vi "Generate VS Channels Info.vi"(11 "Transfer Type":enum16{"Acyclic", "Scheduled"}(ring)) -> (0 "Tx Trigger Channels Array":string[](array[string]), 1 "Tx Disable Channels Array":string[](array[string]), 2 "Tx Channels Array":string[](array[string]), 3 "Rx Channels Array":string[](array[string]), 4 "Is First Parameter? Array":bool[](array[boolean]))   [LabVIEW 2020]
uses:
  b281cc4c-f5bf-4263-a2a4-b8c933cd51f6.vi
  9ae52f1a-1e4b-4aa8-8e73-03c214062afe.vi
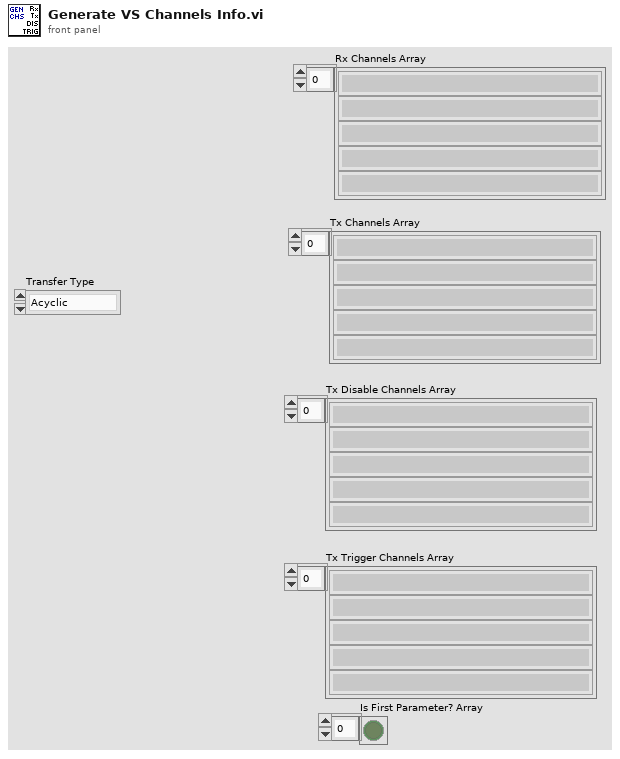
[diagram p1: front panel]
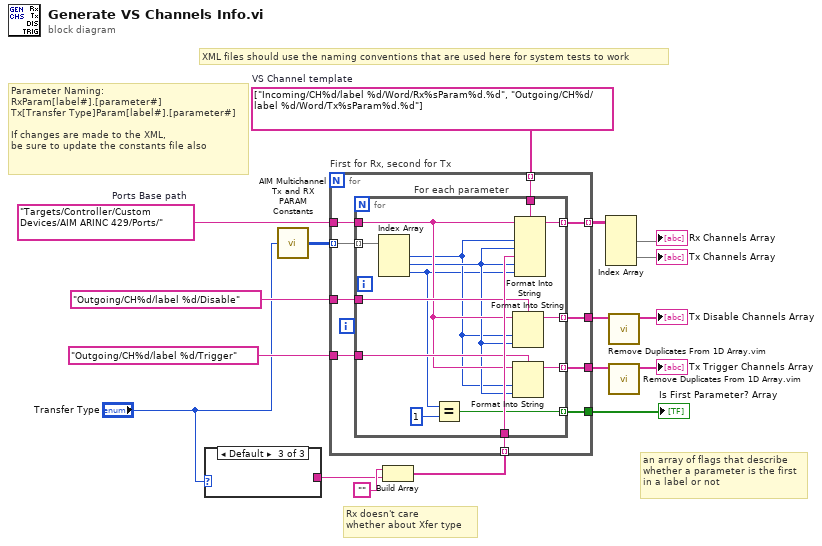
[diagram p0: block diagram]
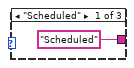
[diagram p2: hidden frame]
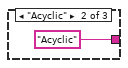
[diagram p3: hidden frame]
diagram:
  w10 = "Targets/Controller/Custom Devices/AIM ARINC 429/Ports/"  # Ports Base path
  w17 = string[] ["Incoming/CH%d/label %d/Word/Rx%sParam%d.%d", "Outgoing/CH%d/label %d/Word/Tx%sParam%d.%d"]  # VS Channel template
  # "Rx doesn't care\nwhether about Xfer type"
  # "an array of flags that describe\nwhether a parameter is the first\nin a label or not"
  # "Parameter Naming:\nRxParam[label#].[parameter#]\nTx[Transfer Type]Param[label#].[parameter#]\n\nIf changes are made to the XML,\nbe sure to update the constants file also"
  # "XML files should use the naming conventions that are used here for system tests to work"
  n1 = case shown="Default" "Transfer Type" {
    tunnel: ["Scheduled" "Acyclic" _] -> w1
    frame "Scheduled" {
    }
    frame "Acyclic" {
    }
    frame Default {
    }
  }
  n2 = call "AIM Multichannel Tx and RX PARAM Constants.vi"("Transfer Type"="Transfer Type") -> ("Parameters (3D Array)"=w9:i32[][][])
  n3 = Build Array("", w1) -> (w4:string[])
  n4 = for "First for Rx, second for Tx" {
    tunnel: [w29] -> w3 mode=indexing
    tunnel: w9 -> [w28] mode=indexing
    tunnel: w10 -> [w27]
    tunnel: w17 -> [w26] mode=indexing
    tunnel: w4 -> [w25] mode=indexing
    tunnel: "Outgoing/CH%d/label %d/Disable" ("String") -> [w24]
    tunnel: [w23] -> w12
    tunnel: "Outgoing/CH%d/label %d/Trigger" ("String") -> [w22]
    tunnel: [w21] -> w14
    tunnel: [w20] -> w8
    n5 = for "For each parameter" {
      tunnel: w28 -> [w43] mode=indexing
      tunnel: w26 -> [w42]
      tunnel: [w41] -> w29 mode=indexing
      tunnel: w27 -> [w36]
      tunnel: w25 -> [w40]
      tunnel: w24 -> [w39]
      tunnel: [w38] -> w23 mode=indexing
      tunnel: w22 -> [w37]
      tunnel: [w34] -> w21 mode=indexing
      tunnel: [w30] -> w20 mode=indexing
      n6 = Index Array(array=w43) -> (element #1=w33:i32, element #2=w35:i32, element #3=w31:i32)  [unwired: 3 in]
      n7 = Equal?(x=w31, y=1) -> (x = y?=w30:bool)
      n8 = Format Into String(format string=w39, initial string=w36, w33, w35) -> (resulting string=w38:string)  [unwired: 1 in, 1 out]
      n9 = Format Into String(format string=w37, initial string=w36, w33, w35) -> (resulting string=w34:string)  [unwired: 1 in, 1 out]
      n10 = Format Into String(format string=w42, initial string=w36, w33, w35, w40, w35, w31) -> (resulting string=w41:string)  [unwired: 1 in, 1 out]
    }
  }
  "Is First Parameter? Array" <- w8
  n11 = Index Array(array=w3) -> (element #1=→"Rx Channels Array":string[], element #2=→"Tx Channels Array":string[])  [unwired: 4 in]
  n12 = call "Remove Duplicates From 1D Array.vim"("array"=w12) -> ("array with duplicates removed"=→"Tx Disable Channels Array":string[])  [unwired: 10 in]
  n13 = call "Remove Duplicates From 1D Array.vim"("array"=w14) -> ("array with duplicates removed"=→"Tx Trigger Channels Array":string[])  [unwired: 10 in]
